vi "Pass Ref and Receive Data.vi"(7 "Enum":T4=enum."Pass Data", 8 "error in (no error)":errorcluster, 10 "Data":T2={"Raw Data"=[], "Volt Channel"={"Index"=[], "Chl Name"=[], "Scale"=[], "Offset"=[], "Sample Rate"=100, "Device Name"="", "Channel"=""}}, 11 "Graph in":refnum<class "Graph.lvclass">) -> (0 "error out":errorcluster, 2 "Data Out":waveform(dbl)[](array[waveform]), 3 "Graph out":refnum<class "Graph.lvclass">)   [LabVIEW 2021, in "Graph.lvclass"]
doc: "This vi has two functions:\nInitialize - Hold This VI Reference in the class\nPass Data - Display data on graph with raw data or conditioned data."
uses:
  Graph.lvclass
  Graph Abstract Class/Pass Ref and Receive Data -- Enum.ctl
  Graph Abstract Class/Graph Data -- cluster.ctl
  Control/Volt Chl.ctl
  Graph Abstract Class/Conditioned Formula  -- Enum.ctl
  Graph.lvclass/Graph.ctl
panel:
  in  "Choose Formula":T1 caption="Choose Formula Applied to the Raw Data"
  out "Waveform Graph":waveform(dbl)[](graph)
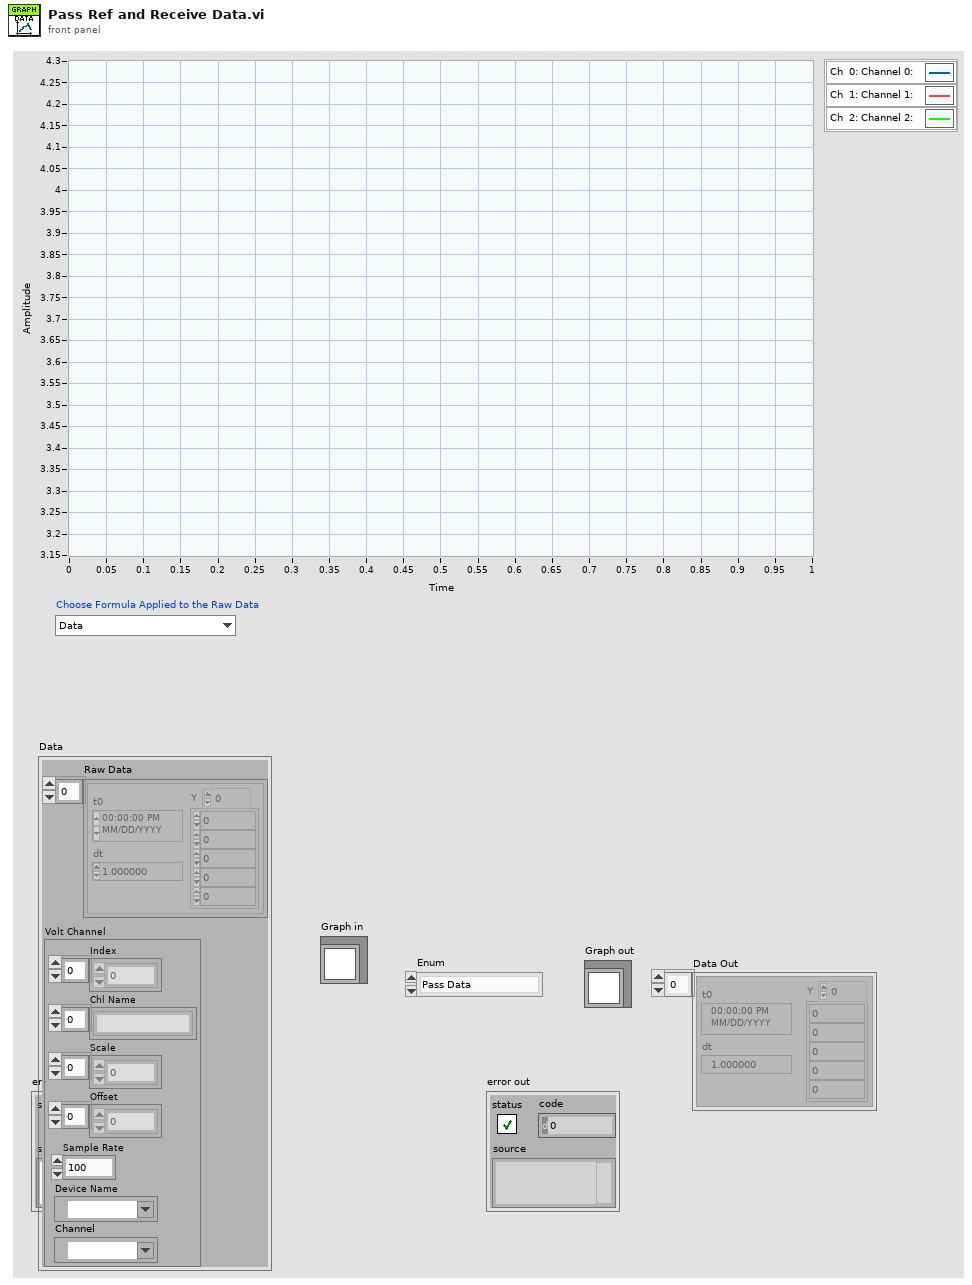
[diagram p1: front panel]
types:
  T1 = typedef "Conditioned Formula  -- Enum.ctl" = enum16{"Data", "Data*Scale+Offset"}
  T2 = typedef "Graph Data -- cluster.ctl" = cluster{"Raw Data":waveform(dbl)[], "Volt Channel":T3}
  T3 = typedef "Volt Chl.ctl" = cluster{"Index":i32[], "Chl Name":string[], "Scale":dbl[], "Offset":dbl[], "Sample Rate":i32, "Device Name":tag, "Channel":tag}
  T4 = typedef "Pass Ref and Receive Data -- Enum.ctl" = enum16{"Initialize", "Pass Data"}
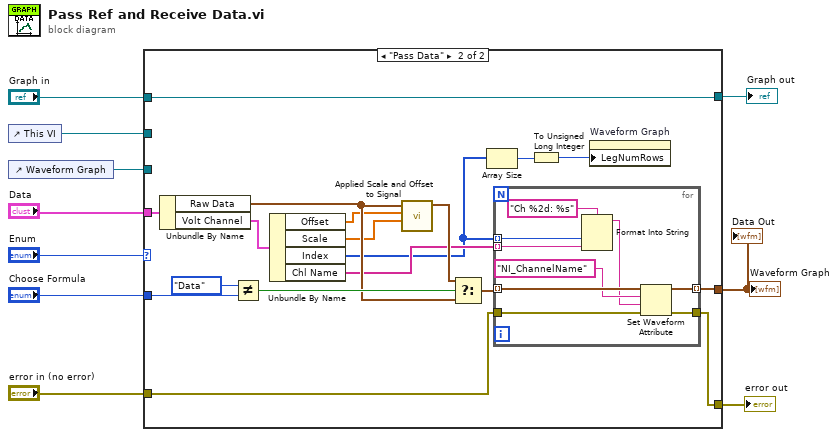
[diagram p0: block diagram]
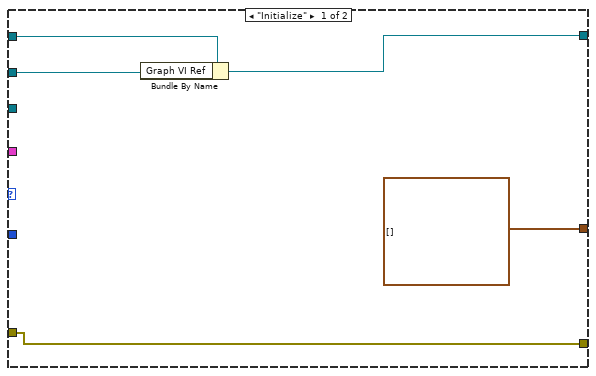
[diagram p2: hidden frame]
diagram:
  n1 = control-ref of="This VI"() -> (w8:refnum<vi>)
  n2 = control-ref of="Waveform Graph"() -> (w6:refnum<vi>)
  n3 = case shown="\"Pass Data\"" "Enum" {
    tunnel: "Data" -> [_ w33]
    tunnel: "Graph in" -> [w15 w32]
    tunnel: [w14 w32] -> w9
    tunnel: w8 -> [w13 _]
    tunnel: w6 -> [_ _]
    tunnel: "Choose Formula" -> [_ w31]
    tunnel: [waveform(dbl)[] [] ("Raw Data") w26] -> w4
    tunnel: "error in (no error)" -> [w11 w24]
    tunnel: [w11 w23] -> w2
    frame "Initialize" {
      n4 = Bundle By Name(cluster=w15, "Graph VI Ref"=w13) -> (w14:refnum<class "Graph.lvclass">)
    }
    frame "Pass Data" {
      n5 = Unbundle By Name(w33) -> ("Raw Data"=w27:waveform(dbl)[], "Volt Channel"=w22:T3)
      n6 = Not Equal?(x=Conditioned_Formula__--_Enum."Data", y=w31) -> (x != y?=w29:bool)
      n7 = Unbundle By Name(w22) -> ("Offset"=w21:dbl[], "Scale"=w20:dbl[], "Index"=w18:i32[], "Chl Name"=w19:string[])
      n8 = call "Applied Scale and Offset to Signal.vi"("Scale"=w20, "Offset"=w21, "Raw Data"=w27) -> ("Conditioned Signal"=w28:waveform(dbl)[])  [unwired: 8 in]
      n9 = Select(t=w28, s=w29, f=w27) -> (s? t:f=w25:waveform(dbl)[])
      n10 = Array Size(array=w18) -> (size(s)=w17:i32)
      n11 = for {
        tunnel: w25 -> [w42] mode=indexing
        tunnel: [w41] -> w26 mode=indexing
        tunnel: w24 -> [w39]
        tunnel: [w38] -> w23
        tunnel: w18 -> [w35] mode=indexing
        tunnel: w19 -> [w34] mode=indexing
        n12 = Format Into String(format string="Ch %2d: %s", w35, w34) -> (resulting string=w36:string)  [unwired: 2 in, 1 out]
        n13 = Set Waveform Attribute(4:w39, 5:w36, 6:"NI_ChannelName" ("name"), 7:w42) -> (0:w38:errorcluster, 3:w41:waveform(dbl))  [unwired: 1 out]
      }
      n14 = To Unsigned Long Integer(number=w17) -> (unsigned 32bit integer=w16:u32)
      n15 = property on="Waveform Graph" class="WFGraph (strict)"("LegNumRows"=w16) -> ()  [unwired: 2 in, 2 out]
    }
  }
  "error out" <- w2
  "Graph out" <- w9
  "Waveform Graph" <- w4
  "Data Out" <- w4
